vi "PID Controller_Autotuning.vi"(0 "output range":cluster{"output high":dbl, "output low":dbl}={"output high"=100.0, "output low"=-100.0} {"output low" format="%.2f"; "output high" format="%.2f"}, 1 "autotuning parameters":T1={"type of controller"=0, "relay cycles"=3, "relay amplitude"=1.0, "control specifications"=2, "PV noise level"=0.1} {"PV noise level" format="%.2f"; "control specifications" items=["normal", "fast", "slow"]; "relay amplitude" format="%.2f"; "type of controller" items=["P", "PI", "PID"]}, 4 "PID gains in":T2={"proportional gain (Kc)"=1.0, "integral time (Ti, min)"=0.01, "derivative time (Td, min)"=0.0} {"derivative time (Td, min)" format="%.3f"; "integral time (Ti, min)" format="%.3f"; "proportional gain (Kc)" format="%.3f"}, 5 "process variable":dbl(slide)=19.583333333333336 scale=0.0..100.0 scale format="%.1f", 6 "dt (s)":dbl=-1.0 format="%.3f", 7 "setpoint":dbl(slide)=30.8641975308642 scale=0.0..100.0 scale format="%.1f", 8 "manipulated variable":dbl(slide)=30.8641975308642 scale=0.0..100.0 scale format="%.1f", 9 "Reinitialize":bool, 10 "Automatic":bool=TRUE, 11 "Autotune":bool) -> (2 "Tuned PID gains":T2={"proportional gain (Kc)"=1.0, "integral time (Ti, min)"=0.01, "derivative time (Td, min)"=0.0} {"derivative time (Td, min)" format="%.3f"; "integral time (Ti, min)" format="%.3f"; "proportional gain (Kc)" format="%.3f"}, 3 "output":dbl format="%.2f")   [LabVIEW 2022 SP3]
uses:
  <vilib>/addons/control/pid/autopid.llb/PID autotuning parameters.ctl
  <vilib>/addons/control/pid/autopid.llb/PID Online Autotuning (Step Closed Loop).vi
  <vilib>/addons/control/pid/pid.llb/PID Advanced (DBL).vi
  <vilib>/addons/control/pid/NI_PID_autopid.lvlib
  <vilib>/addons/control/pid/NI_PID_pid.lvlib
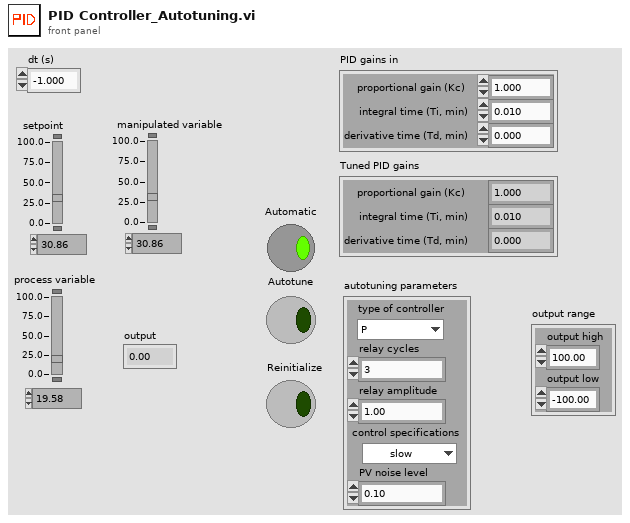
[diagram p1: front panel]
types:
  T1 = typedef "PID autotuning parameters.ctl" = cluster{"type of controller":u16, "relay cycles":i32, "relay amplitude":dbl, "control specifications":u16, "PV noise level":dbl}
  T2 = cluster{"proportional gain (Kc)":dbl, "integral time (Ti, min)":dbl, "derivative time (Td, min)":dbl}
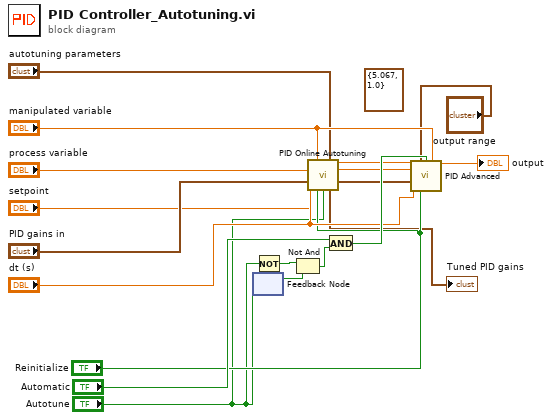
[diagram p0: block diagram]
diagram:
  (unwired) cluster{"output high":dbl, "output low":dbl} {"output high"=5.067, "output low"=1.0} ("output range")
  n1 = feedback #1() -> (w19:bool)  [unwired: 1 in]
  n2 = feedback-in #1("Autotune") -> ()
  n3 = Not(x="Autotune") -> (.not. x?=w18:bool)
  n4 = Not And(1:w19, 2:w18) -> (0:w17:bool)
  n5 = call-poly <vilib>:"PID Online Autotuning.vi"("setpoint"="setpoint", "manipulated variable"="manipulated variable", "autotuning parameters"="autotuning parameters", "process variable"="process variable", "PID gains in"="PID gains in", "dt (s)"="dt (s)", "reinitialize? (F)"="Reinitialize", "autotune? (F)"="Autotune") -> ("setpoint out"=w13:dbl, "process variable out"=w12:dbl, "PID gains out"=w7:T2, "tuned PID gains"=→"Tuned PID gains":T2)  [unwired: 3 in, 1 out]
  n6 = And(x="Automatic", y=w17) -> (x .and. y?=w15:bool)
  n7 = call-poly <vilib>:"PID Advanced.vi"("setpoint"=w13, "output range"="output range", "auto? (T)"=w15, "manual control"="manipulated variable", "process variable"=w12, "PID gains"=w7, "dt (s)"="dt (s)", "reinitialize? (F)"="Reinitialize") -> ("output"=→"output":dbl)  [unwired: 6 in, 1 out]
